vi "LaunchDemo.vi"() -> ()   [LabVIEW 2020]
uses:
  DeviceLoader.vi
panel:
  out "Application Name":string
  out "Waiting Lights":T1
  out "Current Action":string caption="Current action:"
  # "https://sites.psu.edu/hancocklab/"
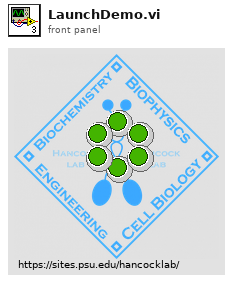
[diagram p1: front panel]
types:
  T1 = cluster{"wait 1":bool, "wait 2":bool, "wait 3":bool, "wait 4":bool, "wait 5":bool, "wait 6":bool}
  T2 = cluster{"[0]":bool, "[1]":bool, "[2]":bool, "[3]":bool, "[4]":bool, "[5]":bool}
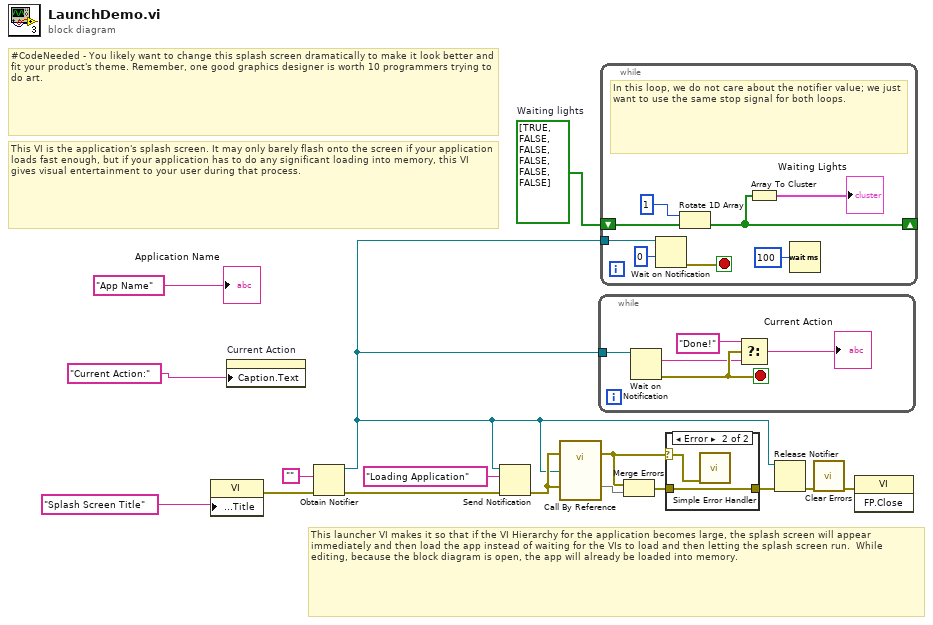
[diagram p0: block diagram]
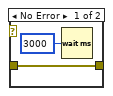
[diagram p2: hidden frame]
diagram:
  w8 = bool[] [TRUE, FALSE, FALSE, FALSE, FALSE, FALSE]  # Waiting lights
  # "#CodeNeeded - You likely want to change this splash screen dramatically to make it look better and fit your product's theme. Remember, one good graphics designer is worth 10 programmers trying to do art."
  # "This VI is the application's splash screen. It may only barely flash onto the screen if your application loads fast enough, but if your application has to do any significant loading into memory, this VI gives visual entertainment to your user during that process."
  # "This launcher VI makes it so that if the VI Hierarchy for the application becomes large, the splash screen will appear immediately and then load the app instead of waiting for the VIs to load and then letting the splash screen run.  While editing, because the block diagram is open, the app will already be loaded into memory."
  n1 = property class="VI"("Front Panel.Title"="Splash Screen Title" ("Window Title")) -> (error out=w16:errorcluster)  [unwired: 2 in, 1 out]
  n2 = property on="Current Action" class="Str"("Caption.Text"="Current Action:" ("Window Title")) -> ()  [unwired: 2 in, 2 out]
  n3 = Obtain Notifier(notification data type="", error in (no error)=w16) -> (notifier out=w11:refnum<notifier>, error out=w6:errorcluster)  [unwired: 2 in, 1 out]
  n4 = Send Notification(notification="Loading Application", notifier=w11, error in (no error)=w6) -> (error out=w12:errorcluster)  [unwired: 1 out]
  n5 = call-by-ref "?"(error in=w12, 1:w11, 4:w12) -> (error out=w2:errorcluster, 18:w15)  [unwired: 17 in, 2 out]
  n6 = while {
    tunnel: w11 -> [w20]
    stop <- w19 stop-if-true
    n7 = Wait on Notification(notifier=w20) -> (notification=w17:string, error out=w19:errorcluster)  [unwired: 3 in, 2 out]
    n8 = Select(t="Done!" ("notification"), s=w19, f=w17) -> (s? t:f=→"Current Action":string)
  }
  n9 = while {
    shift-right: [w23] -> _
    shift-left: w8 -> [w25]
    tunnel: w11 -> [w27]
    stop <- w29 stop-if-true
    # "In this loop, we do not care about the notifier value; we just want to use the same stop signal for both loops."
    n10 = Wait on Notification(notifier=w27, timeout in ms (-1)=0) -> (error out=w29:errorcluster)  [unwired: 2 in, 3 out]
    n11 = Rotate 1D Array(1:w25, 2:1 ("n")) -> (0:w23:bool[])
    n12 = Array To Cluster(array=w23) -> (cluster=→"Waiting Lights":T2)
    n13 = Wait (ms)(milliseconds to wait=u32 100) -> ()  [unwired: 1 out]
  }
  n14 = Merge Errors(w2, w15) -> (w3:errorcluster)
  n15 = case shown="Error" w2 {
    tunnel: [w31 w32] -> w4
    tunnel: w3 -> [w31 w32]
    selector: w2 -> [_ w33]
    frame No Error {
      n16 = Wait (ms)(milliseconds to wait=u32 3000) -> ()  [unwired: 1 out]
    }
    frame Error {
      n17 = call <vilib>:"Simple Error Handler.vi"("error in (no error)"=w33) -> ()  [unwired: 4 in, 5 out]
    }
  }
  n18 = Release Notifier(notifier=w11, error in (no error)=w4) -> (error out=w14:errorcluster)  [unwired: 1 in, 2 out]
  n19 = call <vilib>:"Clear Errors.vi"("error in (no error)"=w14) -> ("error out"=w7:errorcluster)  [unwired: 5 in, 1 out]
  n20 = invoke class="VI" method="FP.Close"(error in=w7) -> ()  [unwired: 2 in, 3 out]
  "Application Name" <- "App Name" ("Unlocalized")
